vi "固件升级（包含参数恢复）.vi"() -> (3 "结果字符串":string)   [LabVIEW 2016, in "斯坦道氨氮.lvlib"]
uses:
  <vilib>/NI/Progress Bar/Controls/Progress Bar Properties.ctl
  <vilib>/NI/Progress Bar/Progress Bar.lvlib
panel:
  out "固件升级步骤":T1
  # "固件升级步骤：\n1、读取固件状态\n2、读取仪器外设设置\n3、读取仪器试剂容量设置\n4、读取仪器量程参数设置\n5、读取仪器公式\n6、写入仪器固件\n7、写入仪器外设设置\n8、写入仪器试剂容量设置\n9、写入仪器量程参数设置\n10、写入仪器公式\n11、询问是否写入流程"
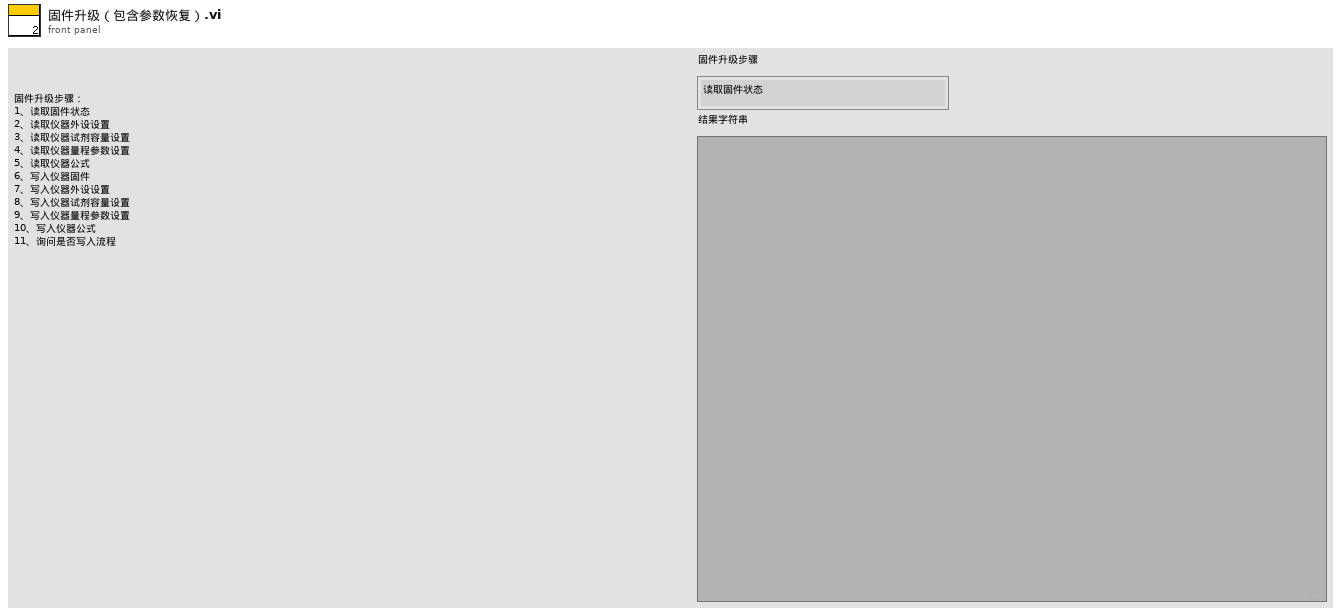
[diagram p1: front panel]
types:
  T1 = typedef "斯坦道氨氮.lvlib/固件升级步骤.ctl" = enum16{"读取固件状态", "读取仪器外设设置", "读取仪器试剂容量设置", "读取仪器量程参数设置", "读取仪器公式", "写入仪器固件", "写入仪器外设设置", "写入仪器试剂容量设置", "写入仪器量程参数", "写入仪器公式", "询问是否写入流程", "写入测试流程", "结束"}
  T2 = typedef "Progress Bar.lvlib/Progress Bar Properties.ctl" = cluster{"Background Color":u32, "Installer Title":string, "Title Color":u32, "Action Text":string, "Text Color":u32, "Slider Value":u8, "Bar Color":u32, "Timeout":i32}
  T3 = cluster{"泵类型":u8, "进样速度":u32, "出样速度":u32, "泵阀量":u8, "光谱仪类型":u8, "光谱采样次数":u8, "氙灯次数":u8, "B":u16, "C":u16, "D":u16, "E":u16, "B_COD":u16, "C_COD":u16, "D_COD":u16, "E_COD":u16, "G":u16, "M":u16, "N":u16, "氨氮注射泵控温下限":sgl, "氨氮注射泵控温上限":sgl, "总氮注射泵控温下限":sgl, "总氮注射泵控温上限":sgl, "消解温度下限":sgl, "消解温度上限":sgl, "加热10s限值":sgl, "高温高压阀开阀温度":sgl, "总氮x公式0":u8, "总氮x公式1":sgl, "总氮x公式2":sgl, "总磷浊度稀释系数":sgl, "总磷浊度补偿权重1":sgl, "总磷浊度补偿权重2":sgl, "盐度系数":sgl, "氨氮补偿系数1":sgl, "氨氮补偿系数2":sgl}
  T4 = cluster{"外设配置":cluster{"泵类型":u8, "进样速度":u32, "出样速度":u32, "泵阀量":u8, "光谱仪类型":u8, "光谱采样次数":u8, "氙灯次数":u8, "B":u16, "C":u16, "D":u16, "E":u16, "B_COD":u16, "C_COD":u16, "D_COD":u16, "E_COD":u16, "G":u16, "M":u16, "N":u16, "氨氮注射泵控温下限":sgl, "氨氮注射泵控温上限":sgl, "总氮注射泵控温下限":sgl, "总氮注射泵控温上限":sgl, "消解温度下限":sgl, "消解温度上限":sgl, "加热10s限值":sgl, "高温高压阀开阀温度":sgl, "总氮x公式0":u8, "总氮x公式1":sgl, "总氮x公式2":sgl, "总磷浊度稀释系数":sgl, "总磷浊度补偿权重1":sgl, "总磷浊度补偿权重2":sgl, "盐度系数":sgl, "氨氮补偿系数1":sgl, "氨氮补偿系数2":sgl}, "error out":errorcluster}
  T5 = cluster{"V1":sgl, "V2":sgl, "V3":sgl, "V4":sgl, "V5":sgl, "V6":sgl, "V7":sgl, "V8":sgl, "V9":sgl, "V10":sgl, "V11":sgl, "V12":sgl, "V9-1":sgl, "V9-2":sgl}
  T6 = cluster{"试剂容量":cluster{"V1":sgl, "V2":sgl, "V3":sgl, "V4":sgl, "V5":sgl, "V6":sgl, "V7":sgl, "V8":sgl, "V9":sgl, "V10":sgl, "V11":sgl, "V12":sgl, "V9-1":sgl, "V9-2":sgl}, "error out":errorcluster}
  T7 = cluster{"测量精度":u16, "检出限":dbl, "上限":dbl, "下限":dbl, "阈值（低->高）":dbl, "阈值（高->低）":dbl, "稀释度":dbl}
  T8 = cluster{"Value":u16, "量程参数读取":cluster{"测量精度":u16, "检出限":dbl, "上限":dbl, "下限":dbl, "阈值（低->高）":dbl, "阈值（高->低）":dbl, "稀释度":dbl}, "error out":errorcluster}
  T9 = cluster{"Value":u16, i32, i32, "公式":cluster{"X^2":dbl, "X":dbl, "b":dbl}, "error out":errorcluster}
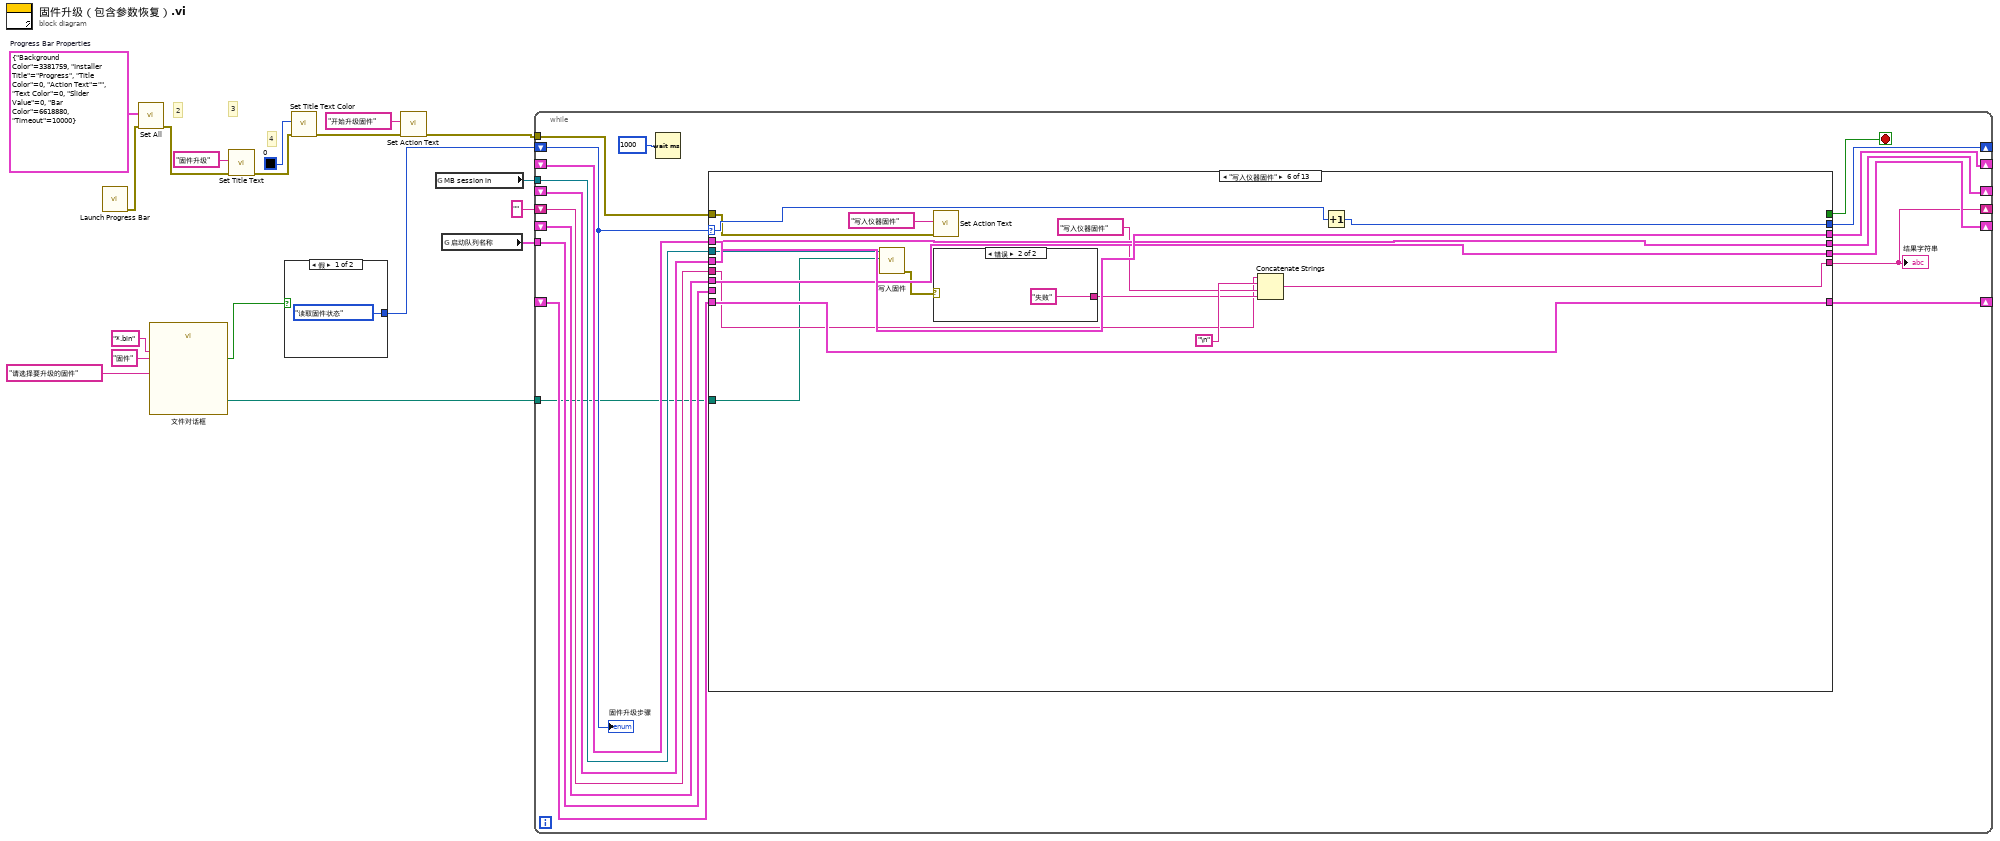
[diagram p0: block diagram]
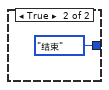
[diagram p2: hidden frame]
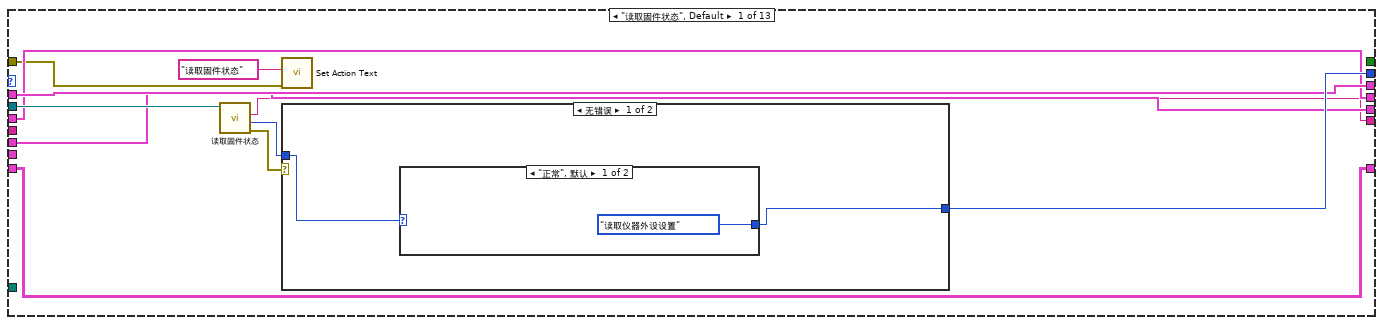
[diagram p3: hidden frame]
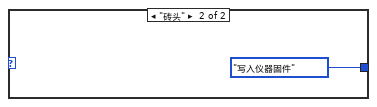
[diagram p4: hidden frame]
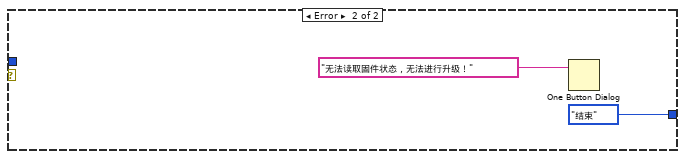
[diagram p5: hidden frame]
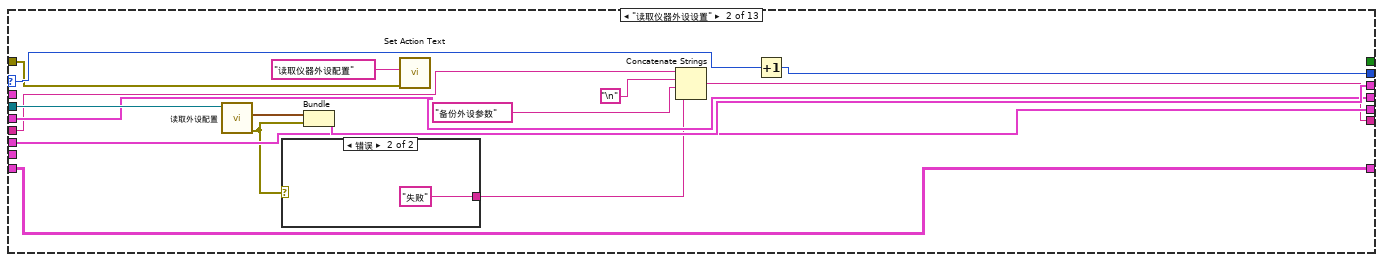
[diagram p6: hidden frame]
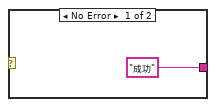
[diagram p7: hidden frame]
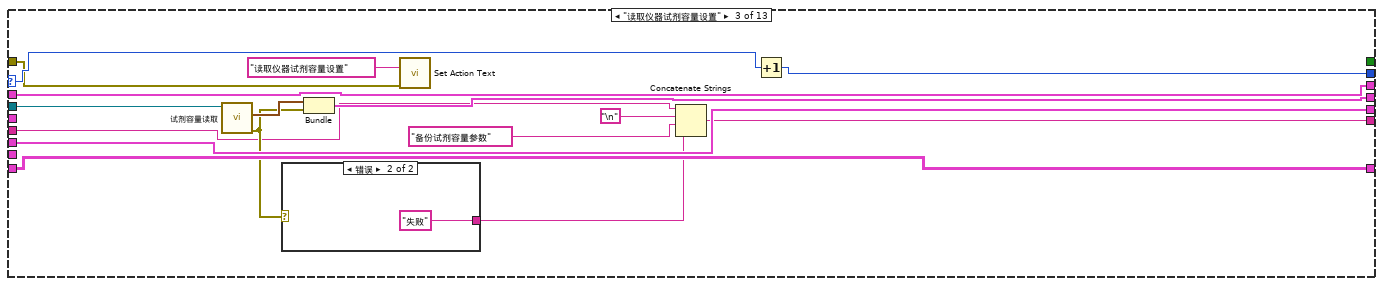
[diagram p8: hidden frame]
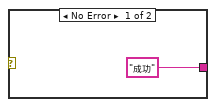
[diagram p9: hidden frame]
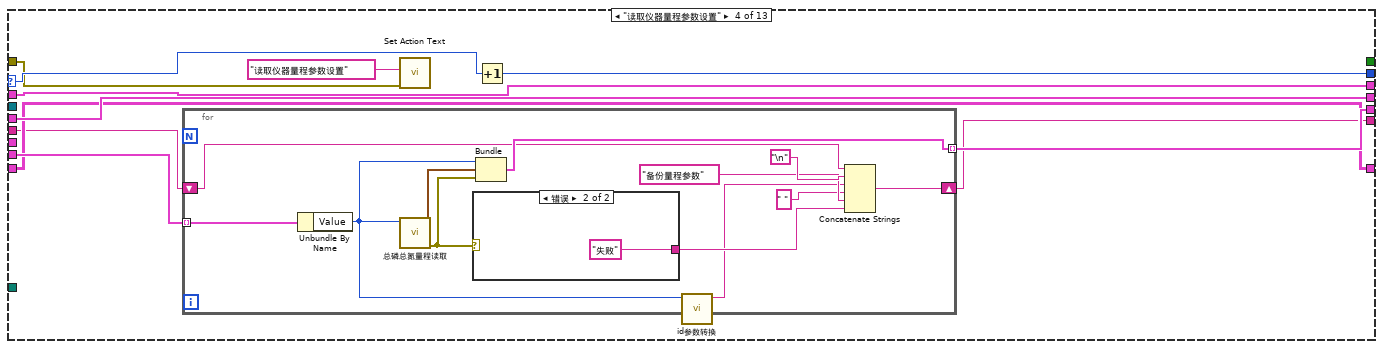
[diagram p10: hidden frame]
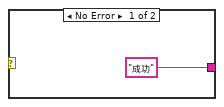
[diagram p11: hidden frame]
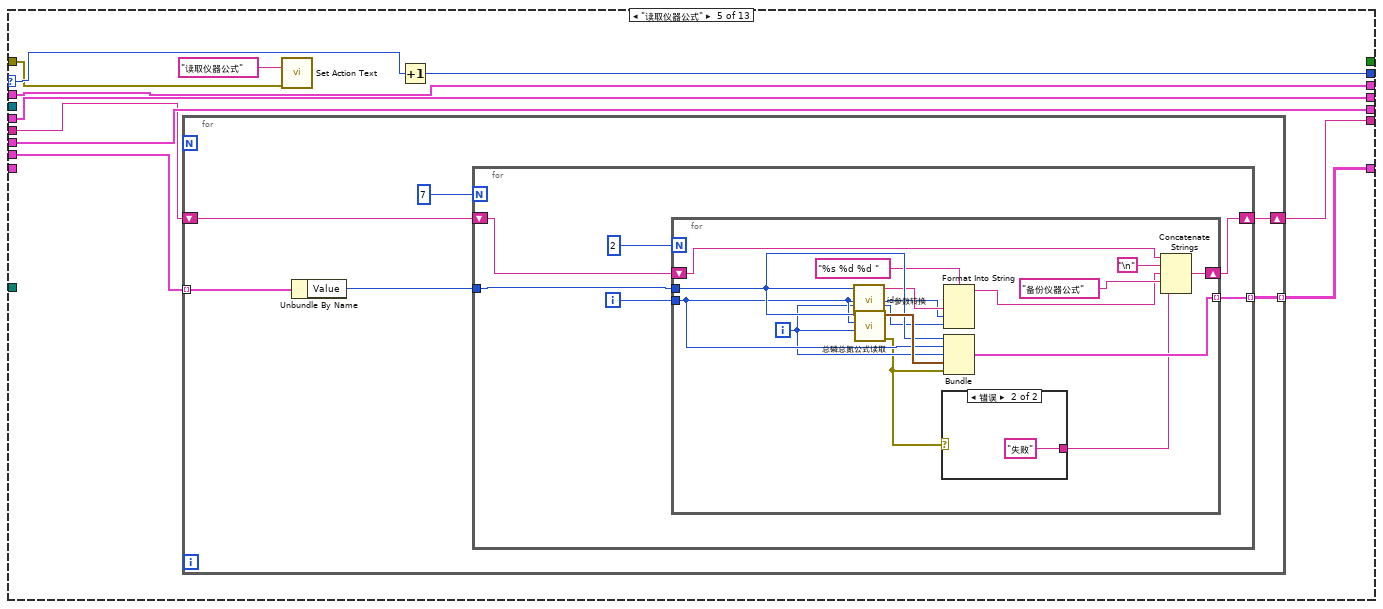
[diagram p12: hidden frame]
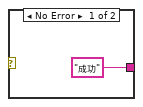
[diagram p13: hidden frame]
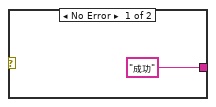
[diagram p14: hidden frame]
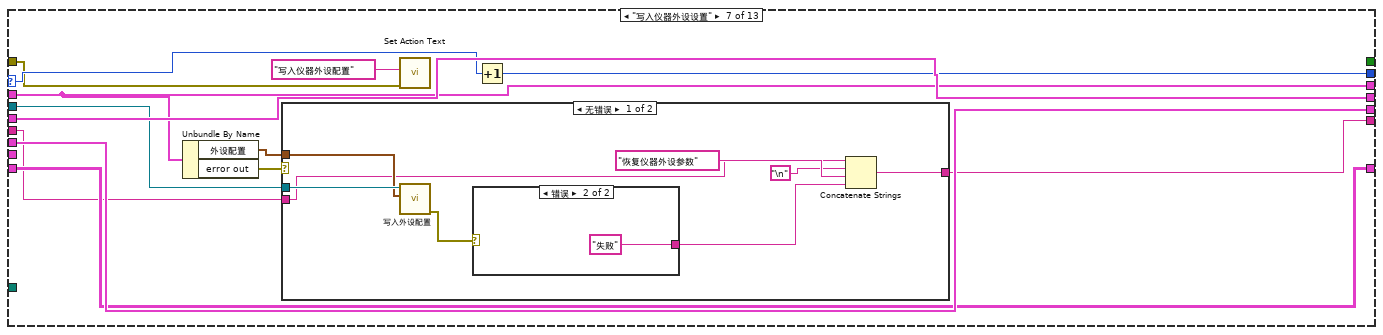
[diagram p15: hidden frame]
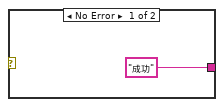
[diagram p16: hidden frame]
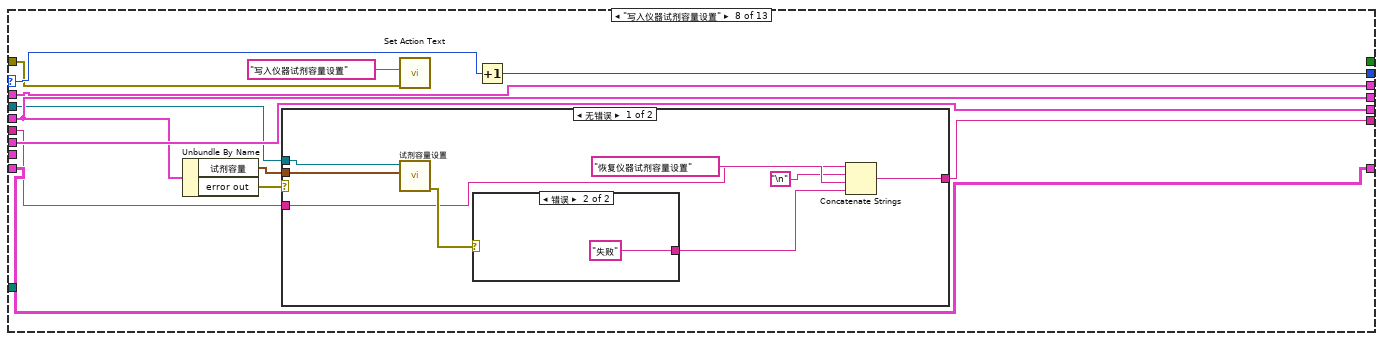
[diagram p18: hidden frame]
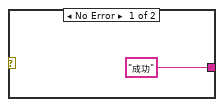
[diagram p19: hidden frame]
diagram:
  w15 = T2 {"Background Color"=3381759, "Installer Title"="Progress", "Title Color"=0, "Action Text"="", "Text Color"=0, "Slider Value"=0, "Bar Color"=6618880, "Timeout"=10000}  # Progress Bar Properties
  # "4"
  # "3"
  # "2"
  n1 = call <vilib>:"Launch Progress Bar.vi"() -> ("error out"=w14:errorcluster)  [unwired: 10 in, 1 out]
  n2 = call <vilib>:"Set All.vi"("error in (no error)"=w14, "Progress Bar Properties (Default)"=w15) -> ("error out"=w11:errorcluster)  [unwired: 9 in]
  n3 = call "文件对话框"("prompt"="请选择要升级的固件", "pattern (all files)"="*.bin", "pattern label"="固件") -> ("selected path"=w3:path, "cancelled"=w2:bool)  [unwired: 9 in, 2 out]
  n4 = call <vilib>:"Set Title Text.vi"("error in (no error)"=w11, "Installer Title"="固件升级") -> ("error out"=w9:errorcluster)  [unwired: 9 in]
  n5 = case shown="假" w2 {
    tunnel: [固件升级步骤."读取固件状态" ("固件升级步骤") 固件升级步骤."结束" ("固件升级步骤")] -> w1
    frame False {
    }
    frame True {
    }
  }
  n6 = call <vilib>:"Set Title Text Color.vi"("error in (no error)"=w9, "Color Box"=u32 0) -> ("error out"=w12:errorcluster)  [unwired: 9 in]
  n7 = call <vilib>:"Set Action Text.vi"("error in (no error)"=w12, "Action Text"="开始升级固件") -> ("error out"=w7:errorcluster)  [unwired: 9 in]
  n8 = global read "VAR总磷总氮全局变量.vi" "MB session in"() -> (w18:refnum<class "MB_Master.lvclass">)
  n9 = global read "总磷总氮断电保存全局变量.vi" "启动队列名称"() -> (w17:cluster{"String":string, "Value":u16}[])
  n10 = while {
    tunnel: w18 -> [w37]
    shift-right: [w36] -> _
    shift-left: w1 -> [w38]
    shift-right: [w34] -> _
    shift-left: _ -> [w33]
    shift-right: [w32] -> _
    shift-left: _ -> [w31]
    tunnel: w17 -> [w30]
    shift-right: [w29] -> _
    shift-left: _ -> [w28]
    shift-right: [w27] -> _
    shift-left: _ -> [w26]
    shift-right: [w23] -> _
    shift-left: "" ("结果字符串") -> [w24]
    tunnel: w7 -> [w22]
    tunnel: w3 -> [w21]
    stop <- w35 stop-if-true
    n11 = Wait (ms)(milliseconds to wait=u32 1000 ("等待时间（毫秒）")) -> ()  [unwired: 1 out]
    n12 = case shown="\"写入仪器固件\"" w38 {
      selector: w38 -> [_ w68 w86 w97 w122 w166 w180 w207 w229 w258 w293 w308 w324]
      tunnel: w37 -> [w49 w71 w89 _ _ w167 w183 w203 _ _ _ _ _]
      tunnel: [w46 w67 w85 w96 w121 w165 w179 w206 w228 w257 w292 w307 w324] -> w36
      tunnel: [_ _ _ _ _ _ _ _ _ _ _ _ TRUE] -> w35
      tunnel: [w45 w69 w84 w100 w125 w171 w182 w210 w231 w260 w299 w314 w323] -> w34
      tunnel: w33 -> [w45 _ w84 w100 w125 w171 w182 w210 w231 w260 w299 w314 w323]
      tunnel: [w44 w66 w87 w99 w124 w170 w186 w205 w227 w259 w298 w313 w322] -> w32
      tunnel: w31 -> [w44 w66 _ w99 w124 w170 w186 w205 w227 w259 w298 w313 w322]
      tunnel: w30 -> [_ _ _ w102 w127 _ _ _ _ _ _ _ _]
      tunnel: [w43 w65 w83 w101 w123 w169 w185 w209 w226 w256 w297 w312 w321] -> w29
      tunnel: w28 -> [w43 w65 w83 _ w123 w169 w185 w209 w226 w256 w297 w312 w321]
      tunnel: [w42 w64 w82 w98 w126 w168 w184 w208 w230 w255 w296 w311 w320] -> w27
      tunnel: w26 -> [w42 w64 w82 w98 _ w168 w184 w208 w230 w255 w296 w311 w320]
      tunnel: [w41 w62 w76 w94 w119 w160 w177 w200 w224 w253 w291 w305 w316] -> w23
      tunnel: w24 -> [_ w61 w77 w95 w120 w161 w176 w201 w225 w254 w291 w306 w317]
      tunnel: w22 -> [w40 w56 w74 w92 w117 w157 w174 w198 w222 w251 _ _ w315]
      tunnel: w21 -> [_ _ _ _ _ w156 _ _ _ _ _ _ _]
      frame "读取固件状态", Default {
        n13 = call "读取固件状态.vi"("MB session in"=w49) -> ("error out"=w47:errorcluster, "固件状态"=w48:enum16{"正常", "砖头"}, "结果字符串"=w41:string)  [unwired: 7 in, 1 out]
        n14 = call <vilib>:"Set Action Text.vi"("error in (no error)"=w40, "Action Text"="读取固件状态") -> ()  [unwired: 9 in, 1 out]
        n15 = case shown="无错误" w47 {
          tunnel: w48 -> [w51 _]
          tunnel: [w50 固件升级步骤."结束" ("固件升级步骤")] -> w46
          frame No Error {
            n16 = case shown="\"正常\", 默认" w51 {
              tunnel: [固件升级步骤."读取仪器外设设置" ("固件升级步骤") 固件升级步骤."写入仪器固件" ("固件升级步骤")] -> w50
              frame "正常", Default {
              }
              frame "砖头" {
              }
            }
          }
          frame Error {
            n17 = One Button Dialog(message="无法读取固件状态，无法进行升级！" ("消息")) -> ()  [unwired: 1 in, 1 out]
          }
        }
      }
      frame "读取仪器外设设置" {
        n18 = call "读取外设配置.vi"("MB session in"=w71) -> ("error out"=w63:errorcluster, "外设配置"=w70:T3)  [unwired: 8 in, 1 out]
        n19 = case shown="错误" w63 {
          tunnel: ["成功" "失败"] -> w59
          frame No Error {
          }
          frame Error {
          }
        }
        n20 = Bundle("外设配置"=w70, "error out"=w63) -> (w69:T4)  [unwired: 1 in]
        n21 = call <vilib>:"Set Action Text.vi"("error in (no error)"=w56, "Action Text"="读取仪器外设配置") -> ()  [unwired: 9 in, 1 out]
        n22 = Concatenate Strings(w61, "\n", "备份外设参数" ("字符串"), w59) -> (w62:string)
        n23 = Increment(x=w68) -> (x+1=w67:T1)
      }
      frame "读取仪器试剂容量设置" {
        n24 = call "试剂容量读取.vi"("MB session in"=w89) -> ("error out"=w78:errorcluster, "试剂容量"=w88:T5)  [unwired: 8 in, 1 out]
        n25 = case shown="错误" w78 {
          tunnel: ["成功" "失败"] -> w80
          frame No Error {
          }
          frame Error {
          }
        }
        n26 = Bundle("试剂容量"=w88, "error out"=w78) -> (w87:T6)  [unwired: 1 in]
        n27 = call <vilib>:"Set Action Text.vi"("error in (no error)"=w74, "Action Text"="读取仪器试剂容量设置") -> ()  [unwired: 9 in, 1 out]
        n28 = Concatenate Strings(w77, "\n", "备份试剂容量参数" ("字符串"), w80) -> (w76:string)
        n29 = Increment(x=w86) -> (x+1=w85:T1)
      }
      frame "读取仪器量程参数设置" {
        n30 = for {
          tunnel: w102 -> [w114] mode=indexing
          tunnel: [w112] -> w101 mode=indexing
          shift-right: [w106] -> w94
          shift-left: w95 -> [w107]
          n31 = Unbundle By Name(w114) -> ("Value"=w105:u16)
          n32 = call "总磷总氮量程读取.vi"("测量参数"=w105) -> ("error out"=w108:errorcluster, "量程参数读取"=w113:T7)  [unwired: 9 in]
          n33 = case shown="错误" w108 {
            tunnel: ["成功" "失败"] -> w110
            frame No Error {
            }
            frame Error {
            }
          }
          n34 = Bundle("Value"=w105, "量程参数读取"=w113, "error out"=w108) -> (w112:T8)  [unwired: 1 in]
          n35 = call "id参数转换.vi"("id"=w105) -> ("table输出"=w104:string)  [unwired: 9 in, 1 out]
          n36 = Concatenate Strings(w107, "\n", w104, " " ("字符串"), "备份量程参数" ("字符串"), w110) -> (w106:string)
        }
        n37 = call <vilib>:"Set Action Text.vi"("error in (no error)"=w92, "Action Text"="读取仪器量程参数设置") -> ()  [unwired: 9 in, 1 out]
        n38 = Increment(x=w97) -> (x+1=w96:T1)
      }
      frame "读取仪器公式" {
        n39 = for {
          tunnel: w127 -> [w133] mode=indexing
          tunnel: [w130] -> w126 mode=indexing
          shift-right: [w128] -> w119
          shift-left: w120 -> [w129]
          n40 = Unbundle By Name(w133) -> ("Value"=w131:u16)
          n41 = for {
            N: 7 -> [_]
            tunnel: w131 -> [w139]
            tunnel: [w136] -> w130 mode=indexing
            shift-right: [w135] -> w128
            shift-left: w129 -> [w134]
            i -> [w138]
            n42 = for {
              N: 2 -> [_]
              tunnel: w139 -> [w146]
              tunnel: w138 -> [w143]
              tunnel: [w152] -> w136 mode=indexing
              shift-right: [w148] -> w135
              shift-left: w134 -> [w147]
              i -> [w142]
              n43 = call "id参数转换.vi"("id"=w146) -> ("table输出"=w144:string)  [unwired: 9 in, 1 out]
              n44 = call "总磷总氮公式读取.vi"("量程"=w142, "测量模式"=w143, "测量参数"=w146) -> ("error out"=w140:errorcluster, "公式"=w153:cluster{"X^2":dbl, "X":dbl, "b":dbl})  [unwired: 7 in]
              n45 = case shown="错误" w140 {
                tunnel: ["成功" "失败"] -> w150
                frame No Error {
                }
                frame Error {
                }
              }
              n46 = Format Into String(format string="%s %d %d " ("格式字符串"), w144, w143, w142) -> (resulting string=w141:string)  [unwired: 2 in, 1 out]
              n47 = Bundle("Value"=w146, w143, w142, "公式"=w153, "error out"=w140) -> (w152:T9)  [unwired: 1 in]
              n48 = Concatenate Strings(w147, "\n", w141, "备份仪器公式" ("字符串"), w150) -> (w148:string)
            }
          }
        }
        n49 = call <vilib>:"Set Action Text.vi"("error in (no error)"=w117, "Action Text"="读取仪器公式") -> ()  [unwired: 9 in, 1 out]
        n50 = Increment(x=w122) -> (x+1=w121:T1)
      }
      frame "写入仪器固件" {
        n51 = call "写入固件.vi"("selected path"=w156, "MB session in"=w167) -> ("error out"=w159:errorcluster)  [unwired: 8 in, 1 out]
        n52 = call <vilib>:"Set Action Text.vi"("error in (no error)"=w157, "Action Text"="写入仪器固件") -> ()  [unwired: 9 in, 1 out]
        n53 = case shown="错误" w159 {
          tunnel: ["成功" "失败"] -> w163
          frame No Error {
          }
          frame Error {
          }
        }
        n54 = Concatenate Strings(w161, "\n", "写入仪器固件" ("字符串"), w163) -> (w160:string)
        n55 = Increment(x=w166) -> (x+1=w165:T1)
      }
      frame "写入仪器外设设置" {
        n56 = Unbundle By Name(w182) -> ("外设配置"=w181:T3, "error out"=w178:errorcluster)
        n57 = case shown="无错误" w178 {
          tunnel: w183 -> [w194 _]
          tunnel: w181 -> [w193 _]
          tunnel: [w188 w197] -> w177
          tunnel: w176 -> [w187 w197]
          frame No Error {
            n58 = call "写入外设配置.vi"("外设配置"=w193, "MB session in"=w194) -> ("error out"=w189:errorcluster)  [unwired: 8 in, 1 out]
            n59 = case shown="错误" w189 {
              tunnel: ["成功" "失败"] -> w191
              frame No Error {
              }
              frame Error {
              }
            }
            n60 = Concatenate Strings(w187, "\n", "恢复仪器外设参数" ("字符串"), w191) -> (w188:string)
          }
          frame Error {
          }
        }
        n61 = call <vilib>:"Set Action Text.vi"("error in (no error)"=w174, "Action Text"="写入仪器外设配置") -> ()  [unwired: 9 in, 1 out]
        n62 = Increment(x=w180) -> (x+1=w179:T1)
      }
      frame "写入仪器试剂容量设置" {
        n63 = Unbundle By Name(w205) -> ("试剂容量"=w204:T5, "error out"=w202:errorcluster)
        n64 = case shown="无错误" w202 {
          tunnel: w204 -> [w218 _]
          tunnel: w203 -> [w217 _]
          tunnel: w201 -> [w212 w221]
          tunnel: [w211 w221] -> w200
          frame No Error {
            n65 = call "试剂容量设置.vi"("试剂容量"=w218, "MB session in"=w217) -> ("error out"=w213:errorcluster)  [unwired: 8 in, 1 out]
            n66 = case shown="错误" w213 {
              tunnel: ["成功" "失败"] -> w215
              frame No Error {
              }
              frame Error {
              }
            }
            n67 = Concatenate Strings(w212, "\n", "恢复仪器试剂容量设置" ("字符串"), w215) -> (w211:string)
          }
          frame Error {
          }
        }
        n68 = call <vilib>:"Set Action Text.vi"("error in (no error)"=w198, "Action Text"="写入仪器试剂容量设置") -> ()  [unwired: 9 in, 1 out]
        n69 = Increment(x=w207) -> (x+1=w206:T1)
      }
      frame "写入仪器量程参数" {
        n70 = for {
          tunnel: w226 -> [w237] mode=indexing
          shift-right: [w232] -> w224
          shift-left: w225 -> [w233]
          n71 = Unbundle By Name(w237) -> ("Value"=w235:u16, "量程参数读取"=w236:T7, "error out"=w234:errorcluster)
          n72 = case shown="无错误" w234 {
            tunnel: w236 -> [w247 _]
            tunnel: w235 -> [w240 _]
            tunnel: w233 -> [w242 w250]
            tunnel: [w241 w250] -> w232
            frame No Error {
              n73 = call "总磷总氮量程写入.vi"("量程参数写入"=w247, "测量参数"=w240) -> ("error out"=w243:errorcluster)  [unwired: 8 in]
              n74 = case shown="错误" w243 {
                tunnel: ["成功" "失败"] -> w245
                frame No Error {
                }
                frame Error {
                }
              }
              n75 = call "id参数转换.vi"("id"=w240) -> ("table输出"=w239:string)  [unwired: 9 in, 1 out]
              n76 = Concatenate Strings(w242, "\n", w239, " " ("字符串"), "恢复仪器量程参数" ("字符串"), w245) -> (w241:string)
            }
            frame Error {
            }
          }
        }
        n77 = call <vilib>:"Set Action Text.vi"("error in (no error)"=w222, "Action Text"="写入仪器量程参数设置") -> ()  [unwired: 9 in, 1 out]
        n78 = Increment(x=w229) -> (x+1=w228:T1)
      }
      frame "写入仪器公式" {
        n79 = for {
          tunnel: w255 -> [w263] mode=indexing
          shift-right: [w261] -> w253
          shift-left: w254 -> [w262]
          n80 = for {
            tunnel: w263 -> [w266] mode=indexing
            shift-right: [w264] -> w261
            shift-left: w262 -> [w265]
            n81 = for {
              tunnel: w266 -> [w274] mode=indexing
              shift-right: [w267] -> w264
              shift-left: w265 -> [w268]
              n82 = Unbundle(w274) -> ("Value"=w272:u16, w271:i32, w270:i32, "公式"=w269:cluster{"X^2":dbl, "X":dbl, "b":dbl}, "error out"=w273:errorcluster)
              n83 = case shown="无错误" w273 {
                tunnel: w272 -> [w279 _]
                tunnel: w271 -> [w278 _]
                tunnel: w270 -> [w277 _]
                tunnel: w269 -> [w287 _]
                tunnel: w268 -> [w276 w290]
                tunnel: [w275 w290] -> w267
                frame No Error {
                  n84 = call "总磷总氮公式写入.vi"("公式"=w287, "量程"=w277, "测量模式"=w278, "测量参数"=w279) -> ("error out"=w280:errorcluster)  [unwired: 7 in]
                  n85 = case shown="错误" w280 {
                    tunnel: ["成功" "失败"] -> w285
                    frame No Error {
                    }
                    frame Error {
                    }
                  }
                  n86 = call "id参数转换.vi"("id"=w279) -> ("table输出"=w282:string)  [unwired: 9 in, 1 out]
                  n87 = Format Into String(format string="%s %d %d " ("格式字符串"), w282, w278, w277) -> (resulting string=w281:string)  [unwired: 2 in, 1 out]
                  n88 = Concatenate Strings(w276, "\n", w281, "恢复仪器公式" ("字符串"), w285) -> (w275:string)
                }
                frame Error {
                }
              }
            }
          }
        }
        n89 = call <vilib>:"Set Action Text.vi"("error in (no error)"=w251, "Action Text"="写入仪器公式") -> ()  [unwired: 9 in, 1 out]
        n90 = Increment(x=w258) -> (x+1=w257:T1)
      }
      frame "询问是否写入流程" {
        n91 = Two Button Dialog(message="是否写入流程" ("消息")) -> (T button?=w294:bool)  [unwired: 2 in]
        n92 = case shown="假" w294 {
          tunnel: w293 -> [_ w302]
          tunnel: [固件升级步骤."结束" w301] -> w292
          frame False {
          }
          frame True {
            n93 = Increment(x=w302) -> (x+1=w301:T1)
          }
        }
      }
      frame "写入测试流程" {
        n94 = Concatenate Strings(w306, "\n", "写入流程" ("字符串")) -> (w305:string)
        n95 = global read "总磷总氮断电保存全局变量.vi" "简易流程路径"() -> (w309:path)
        n96 = global read "总磷总氮断电保存全局变量.vi" "流程路径"() -> (w310:path)
        n97 = call "流程写入.vi"("简易流程路径"=w309, "添加的路径"=w310) -> ()  [unwired: 10 in]
        n98 = Increment(x=w308) -> (x+1=w307:T1)
      }
      frame "结束" {
        n99 = call <vilib>:"Close Progress Bar.vi"("error in (no error)"=w315) -> ()  [unwired: 9 in, 2 out]
        n100 = Concatenate Strings(w317, "\n", "结束" ("字符串")) -> (w316:string)
      }
    }
    "结果字符串" <- w23
    "固件升级步骤" <- w38
  }
